vi "Write TEC.vi"(8 "error in (no error)":errorcluster, 10 "TEC":refnum<vi>, 11 "TEC Controller in":refnum<class "TEC Controller.lvclass">) -> (0 "error out":errorcluster, 3 "TEC Controller out":refnum<class "TEC Controller.lvclass">)   [LabVIEW 2014, in "Humidifier Test Lib.lvlib" / "TEC Controller.lvclass"]
uses:
  TEC Controller.lvclass
  TEC Controller.lvclass/TEC Controller.ctl
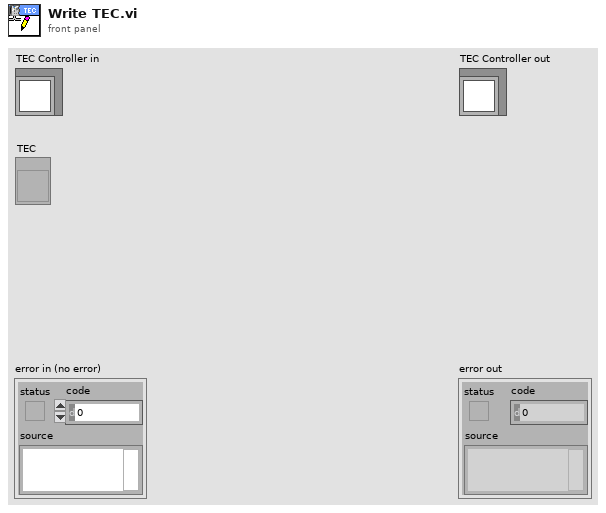
[diagram p1: front panel]
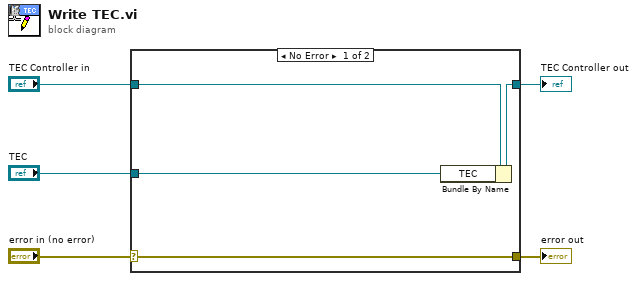
[diagram p0: block diagram]
diagram:
  n1 = case shown="No Error" "error in (no error)" {
    selector: "error in (no error)" -> [w9 w10]
    tunnel: [w9 w10] -> w4
    tunnel: [w7 w11] -> w2
    tunnel: "TEC Controller in" -> [w8 w11]
    tunnel: "TEC" -> [w6 _]
    frame No Error {
      n2 = Bundle By Name(cluster=w8, "TEC"=w6) -> (w7:refnum<class "TEC Controller.lvclass">)
    }
    frame Error {
    }
  }
  "error out" <- w4
  "TEC Controller out" <- w2
